vi "CONTROLE DE TEMPERATURA.vi"() -> ()   [LabVIEW 2019]
uses:
  ctl's/state machine.ctl
  <vilib>/Platform/TimedLoop/XDataNode/timing_clust.ctl
  <vilib>/Platform/TimedLoop/XDataNode/nitl_modes.ctl
  <vilib>/Platform/TimedLoop/XDataNode/wakeup.ctl
  <vilib>/platform/TimedLoop/XDataNode/XDataNode.xnode
  <vilib>/Platform/TimedLoop/XDataNode/XDNodeRunTimeDep.lvlib
panel:
  out "INFORMATIONS":T2 {"Temperature" scale=15.0..40.0}
  out "Temperature Graph":dbl(graph)
  in  "stop":bool
  in  "OFF/ ON":bool
  # "FINITE STATE MACHINE"
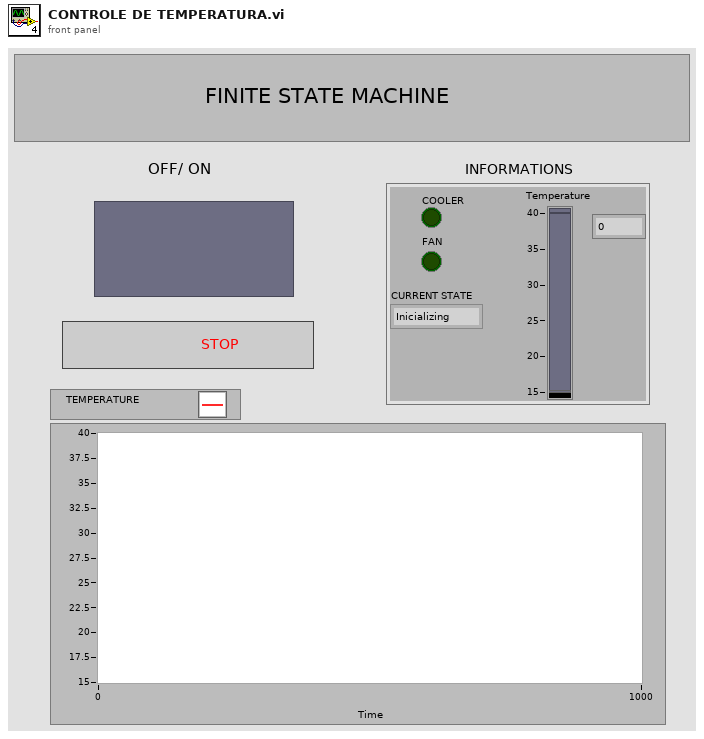
[diagram p1: front panel]
types:
  T1 = typedef "state machine.ctl" = enum16{"Inicializing", "Fan", "Fan + cooler", "cooler", "OFF", "Heating"}
  T2 = cluster{"COOLER":bool, "FAN":bool, "CURRENT STATE":T1, "Temperature":dbl}
  T3 = typedef "XDNodeRunTimeDep.lvlib/timing_clust.ctl" = cluster{"Expected End [f-1]":u64, "Actual End [f-1]":u64, "Finished Late? [f-1]":bool, "Expected End [i-1]":u64, "Actual End [i-1]":u64, "Finished Late? [i-1]":bool, "Expected Start [i]":u64, "Actual Start [i]":u64, "Expected Start [f]":u64, "Actual Start [f]":u64, "Source Name":string, "Structure Name":string, "Period":i64, "Deadline":i64, "Offset":i64, "Start":i64, "Priority":i32, "Timeout":i32, "Mode":T4, "Wakeup Reason":T5, "Error":errorcluster, "Source Type":string, "Secondary Source Type":string, "Global End Time":u64, "Global Start Time":u64, "Frame Duration":u64, "Iteration Duration":u64, "Assigned CPU":i32, "I/O Scan Engine Mode":u32}
  T4 = typedef "XDNodeRunTimeDep.lvlib/nitl_modes.ctl" = enum32{"No Change", "Process missed periods, maintain original phase", "Discard missed periods, maintain original phase", "Process missed periods, ignore original phase", "Discard missed periods, ignore original phase"}
  T5 = typedef "XDNodeRunTimeDep.lvlib/wakeup.ctl" = enum32{"Normal", "Aborted", "Asynchronous wakeup", "Timing source error", "Timed loop error", "Timeout"}
  T6 = cluster{"COOLER":bool, "VENTILADOR":bool, "Estado atual":T1, "Temperatura":dbl}
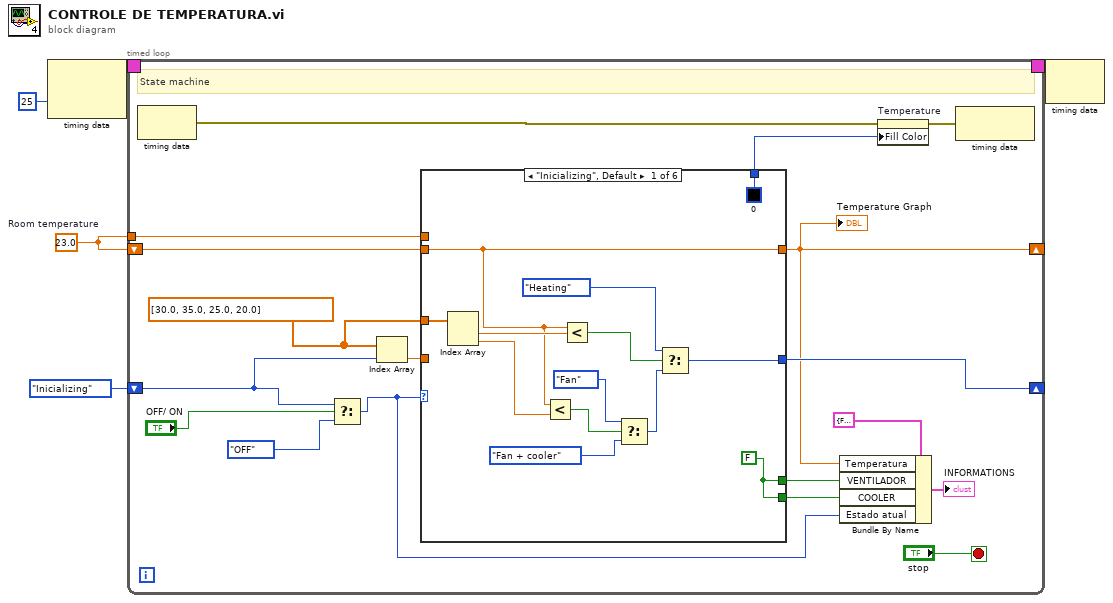
[diagram p0: block diagram]
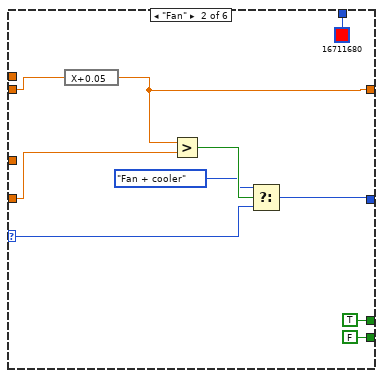
[diagram p2: hidden frame]
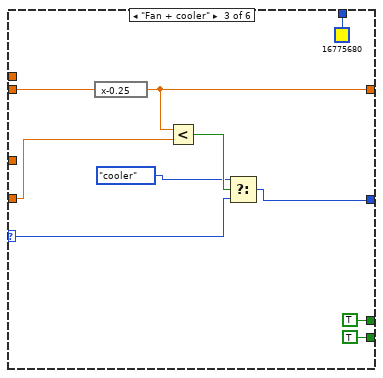
[diagram p3: hidden frame]
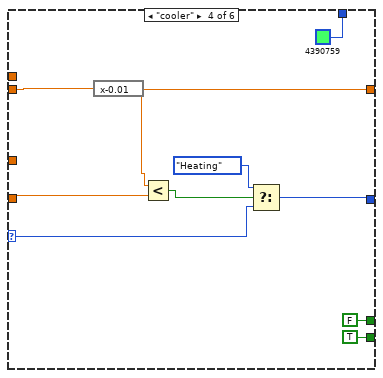
[diagram p4: hidden frame]
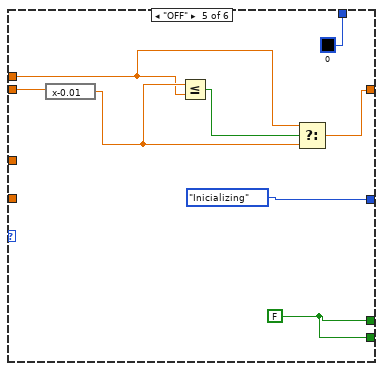
[diagram p5: hidden frame]
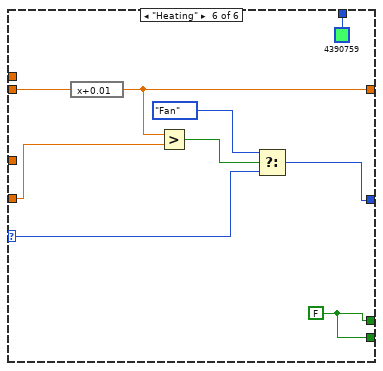
[diagram p6: hidden frame]
diagram:
  w1 = 23.0  # Room temperature
  n1 = node-c288(i64 25 ("Period")) -> (w5:T3)  [unwired: 1 in]
  n2 = timed-loop {
    timing: w5 -> [_]
    timing-out: [_] -> w4
    shift-right: [w15] -> _
    shift-left: state_machine."Inicializing" -> [w21]
    shift-right: [w9] -> _
    shift-left: w1 -> [w18]
    tunnel: w1 -> [w14]
    stop <- "stop" stop-if-true
    w20 = dbl[] [30.0, 35.0, 25.0, 20.0] ("array")
    # "State machine"
    n3 = node-c288() -> (w8:errorcluster)  [unwired: 1 in]
    n4 = Select(t=w21, s="OFF/ ON", f=state_machine."OFF") -> (s? t:f=w12:T1)
    n5 = Index Array(array=w20, index=w21) -> (element=w19:dbl)
    n6 = case shown="\"Inicializing\", Default" w12 {
      selector: w12 -> [_ w41 w51 w59 _ w77]
      tunnel: w20 -> [w36 _ _ _ _ _]
      tunnel: w19 -> [_ w46 w54 w61 _ w80]
      tunnel: w18 -> [w26 w38 w56 w66 w74 w82]
      tunnel: [w25 w43 w50 w58 state_machine."Inicializing" w76] -> w15
      tunnel: [w27 TRUE TRUE FALSE w73 w83] -> w17
      tunnel: [w27 FALSE TRUE TRUE w73 w83] -> w16
      tunnel: [w26 w44 w55 w62 w72 w81] -> w9
      tunnel: w14 -> [_ _ _ _ w69 _]
      tunnel: [u32 0 ("Fill Color") u32 16711680 ("Fill Color") u32 16775680 ("Fill Color") u32 4390759 ("Fill Color") u32 0 ("Fill Color") u32 4390759 ("Fill Color")] -> w6
      frame "Inicializing", Default {
        w27 = FALSE
        n7 = Index Array(array=w36) -> (element #1=w35:dbl, element #2=w34:dbl)  [unwired: 2 in]
        n8 = Less?(x=w26, y=w34) -> (x < y?=w33:bool)
        n9 = Less?(x=w26, y=w35) -> (x < y?=w32:bool)
        n10 = Select(t=state_machine."Fan", s=w33, f=state_machine."Fan + cooler") -> (s? t:f=w29:T1)
        n11 = Select(t=state_machine."Heating", s=w32, f=w29) -> (s? t:f=w25:T1)
      }
      frame "Fan" {
        n12 = expression code="X+0.05"(w38) -> (w44:dbl)
        n13 = Greater?(x=w44, y=w46) -> (0:w45:bool)
        n14 = Select(t=state_machine."Fan + cooler", s=w45, f=w41) -> (s? t:f=w43:T1)
      }
      frame "Fan + cooler" {
        n15 = expression code="x-0.25"(w56) -> (w55:dbl)
        n16 = Less?(x=w55, y=w54) -> (x < y?=w53:bool)
        n17 = Select(t=state_machine."cooler", s=w53, f=w51) -> (s? t:f=w50:T1)
      }
      frame "cooler" {
        n18 = expression code="x-0.01"(w66) -> (w62:dbl)
        n19 = Less?(x=w62, y=w61) -> (x < y?=w63:bool)
        n20 = Select(t=state_machine."Heating", s=w63, f=w59) -> (s? t:f=w58:T1)
      }
      frame "OFF" {
        w73 = FALSE
        n21 = expression code="x-0.01"(w74) -> (w70:dbl)
        n22 = Less Or Equal?(x=w70, y=w69) -> (x <= y?=w68:bool)
        n23 = Select(t=w69, s=w68, f=w70) -> (s? t:f=w72:dbl)
      }
      frame "Heating" {
        w83 = FALSE
        n24 = expression code="x+0.01"(w82) -> (w81:dbl)
        n25 = Greater?(x=w81, y=w80) -> (0:w79:bool)
        n26 = Select(t=state_machine."Fan", s=w79, f=w77) -> (s? t:f=w76:T1)
      }
    }
    "Temperature Graph" <- w9
    n27 = Bundle By Name(cluster=T6 {"COOLER"=FALSE, "VENTILADOR"=FALSE, "Estado atual"=enum."Inicializing", "Temperatura"=0.0} ("Cluster"), "Temperatura"=w9, "VENTILADOR"=w17, "COOLER"=w16, "Estado atual"=w12) -> (→"INFORMATIONS":T6)
    n28 = property on="Temperature" class="Slide (strict)"(error in=w8, "Fill Color"=w6) -> (error out=w7:errorcluster)  [unwired: 1 in, 1 out]
    n29 = node-c288(w7) -> ()  [unwired: 1 out]
  }
  n30 = node-c288(w4) -> ()  [unwired: 1 out]
